vi "Query DUT Connector Band Catalog.vi"(8 "error in (no error)":errorcluster, 9 "Connector (\"Connector1\")":string="Connector1", 10 "DUT (\"DUT1\")":string="DUT1", 11 "VISA resource name":refnum<visa-resource-name>) -> (0 "error out":errorcluster, 2 "Connector Bands":string, 3 "VISA resource name out":refnum<visa-resource-name>)   [LabVIEW 2020, in "Rohde&Schwarz CMXP Base.lvlib"]
doc: "Queries a list of all frequency bands assigned to an antenna connector of the inactive DUT <DutName>. The command is structured according to the connector-centric approach.\n\nThe results are returned as groups of values, with <NoOfBands> pairs of <RatType>, <BandNumber> per group:\n\n{<TX>, <RX>, <NoOfBands>, {<RatType>, <BandNumber>,}<NoOfBands> times} ...\n\nAttribute:\n-\n\nRemote-control command:\nCATalog:DUT:PROFile:CONNector:BAND?"
uses:
  <instrlib>/Rohde&Schwarz CMXP Base/Rohde&Schwarz CMXP Base.lvlib
  <instrlib>/Rohde&Schwarz CMXP Base/Private/rsidr_core.llb/rsidr_core.lvlib
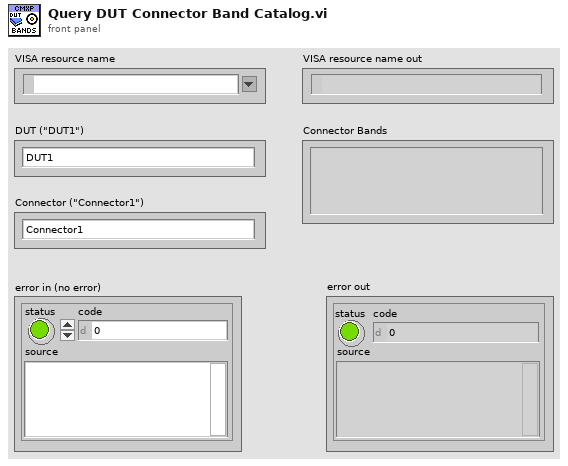
[diagram p1: front panel]
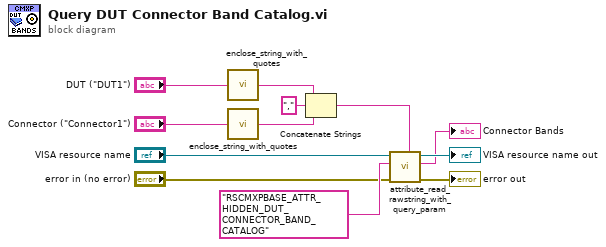
[diagram p0: block diagram]
diagram:
  n1 = call <instrlib>:"enclose_string_with_quotes.vi"("String to enclose"="DUT (\"DUT1\")") -> ("String out"=w3:string)  [unwired: 4 in]
  n2 = call <instrlib>:"enclose_string_with_quotes.vi"("String to enclose"="Connector (\"Connector1\")") -> ("String out"=w4:string)  [unwired: 4 in]
  n3 = Concatenate Strings(w3, "," ("string"), w4) -> (w1:string)
  n4 = call <instrlib>:"attribute_read_rawstring_with_query_param.vi"("Query Parameter (None)"=w1, "error in"="error in (no error)", "Attribute ID"="RSCMXPBASE_ATTR_HIDDEN_DUT_CONNECTOR_BAND_CATALOG", "VISA resource name"="VISA resource name") -> ("error out"=→"error out":errorcluster, "RawString out"=→"Connector Bands":string, "VISA resource name out"=→"VISA resource name out":refnum<visa-resource-name>)  [unwired: 5 in]
